vi "Creator.vi"(9 "Priority?":bool, 10 "Msg Strategy":refnum<class "Msg Strategy.lvclass">, 11 "TEMPLATE jettl in":refnum<class "TEMPLATE jettl.lvclass">) -> (3 "TEMPLATE jettl out":refnum<class "TEMPLATE jettl.lvclass">)   [LabVIEW 2021, in "_Template.lvlib" / "Templates.lvlib" / "TEMPLATE jettl.lvlib" / "TEMPLATE jettl.lvclass"]
uses:
  TEMPLATE jettl.lvclass
  jettl/jettl/Msg Strategy/Msg Strategy.lvclass
  TEMPLATE jettl.lvclass/TEMPLATE jettl.ctl
  jettl/jettl/jettl/jettl.lvclass
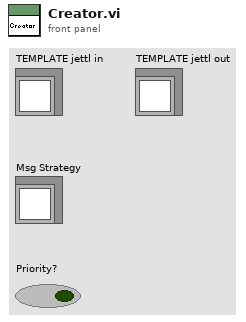
[diagram p1: front panel]
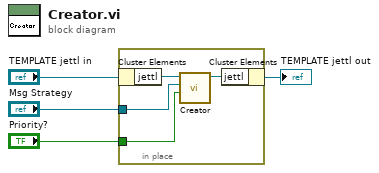
[diagram p0: block diagram]
diagram:
  n1 = in-place {
    in-place-border: "Msg Strategy" -> [w6]
    in-place-border: "Priority?" -> [w5]
    n2 = in-place-cluster #1("TEMPLATE jettl in") -> ("jettl"=w8:refnum<class "jettl.lvclass">)
    n3 = call-dynamic "Creator.vi"("Priority?"=w5, "Msg Strategy"=w6, "jettl in"=w8) -> ("jettl out"=w7:refnum<class "jettl.lvclass">)  [unwired: 8 in]
    n4 = in-place-cluster #1("jettl"=w7) -> (→"TEMPLATE jettl out":refnum<class "TEMPLATE jettl.lvclass">)
  }
